vi "Log Sequence FGV.vi"(6 "Aktion":T3, 9 "Neue Gasliste gesamt":T1[](array[typedef]), 11 "Cluster (in)":T2) -> (3 "Cluster (out)":T2)   [LabVIEW 2020, in "LogKonfig.lvlib"]
uses:
  Log Sequence FGV Aktion.ctl
  Visualisierungs Elemente/String - Ausgabefeld.ctl
  LogKonfig.lvlib
  AK-Schnittstelle/AK-Schnittstelle.lvlib
  Allgemein/allgemeine Sub-VIs.lvlib
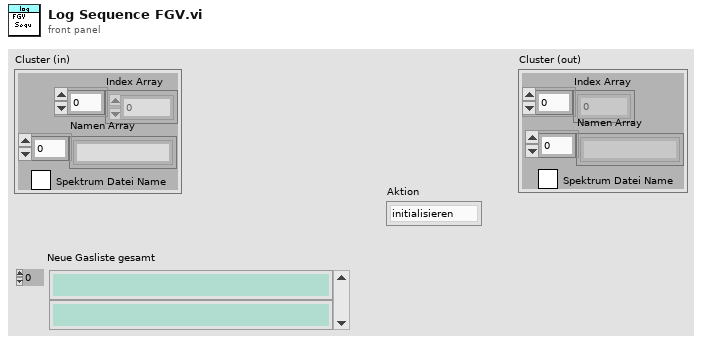
[diagram p1: front panel]
types:
  T1 = typedef "String - Ausgabefeld.ctl" = string
  T2 = cluster{"Index Array":i32[], "Namen Array":string[], "Spektrum File Name":bool}
  T3 = typedef "LogKonfig.lvlib/Log Sequence FGV Aktion.ctl" = enum16{"initialisieren", "lesen", "schreiben", "laden", "speichern", "übertragen"}
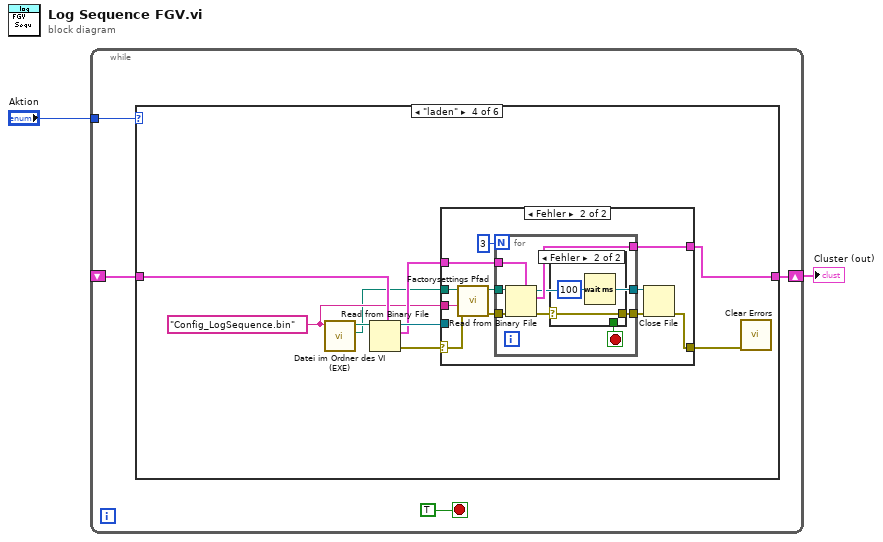
[diagram p0: block diagram]
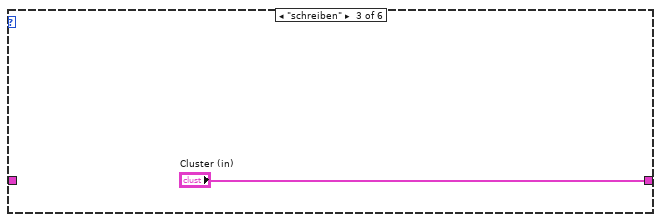
[diagram p4: hidden frame]
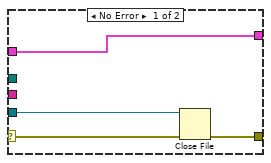
[diagram p5: hidden frame]
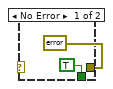
[diagram p6: hidden frame]
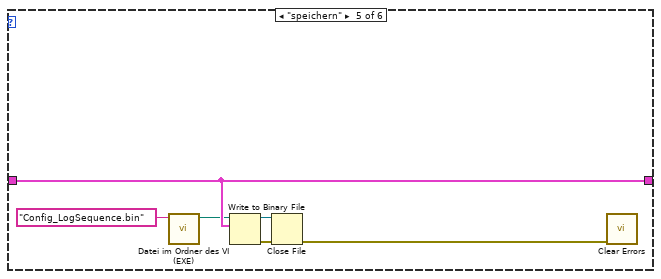
[diagram p7: hidden frame]
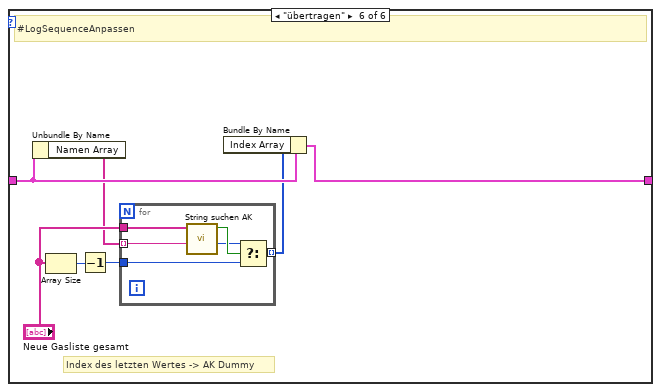
[diagram p8: hidden frame]
diagram:
  n1 = while {
    tunnel: "Aktion" -> [w5]
    shift-right: [w4] -> w1
    shift-left: _ -> [w3]
    stop <- TRUE stop-if-true
    n2 = case shown="\"laden\"" w5 {
      tunnel: [_ w7 "Cluster (in)" w13 w50 w56] -> w4
      tunnel: w3 -> [_ w7 _ w17 w50 w57]
      frame "initialisieren", Default {
      }
      frame "lesen" {
      }
      frame "schreiben" {
      }
      frame "laden" {
        w10 = "Config_LogSequence.bin" ("Dateiname")
        n3 = call "Datei im Ordner des VI (EXE).vi"("Dateiname"=w10) -> ("Ordner des Haupt-VIs"=w9:path, "Dateipfad im Ordner des Haupt-VIs"=w11:path)  [unwired: 8 in, 1 out]
        n4 = Read from Binary File(5:w17, 11:w11) -> (0:w15:errorcluster, 2:w14:T2, 3:w16:refnum<file>)  [unwired: 4 in, 1 out]
        n5 = case shown="Fehler" w15 {
          selector: w15 -> [w20 w24]
          tunnel: w14 -> [w21 w27]
          tunnel: [w21 w31] -> w13
          tunnel: [w18 w29] -> w12
          tunnel: w16 -> [w19 _]
          tunnel: w9 -> [_ w23]
          tunnel: w10 -> [_ w22]
          frame No Error {
            n6 = Close File(refnum=w19, error in=w20) -> (error out=w18:errorcluster)  [unwired: 1 out]
          }
          frame Error {
            n7 = call "Factorysettings Pfad.vi"("error in (no error)"=w24, "Dateiname"=w22, "Ordner des Haupt-VIs"=w23) -> ("error out"=w25:errorcluster, "Pfad Factorysettings"=w26:path)  [unwired: 7 in]
            n8 = for {
              N: 3 -> [_]
              tunnel: w25 -> [w38]
              tunnel: w26 -> [w37]
              tunnel: [w36] -> w31
              tunnel: [w35] -> w30
              tunnel: [w34] -> w28
              tunnel: w27 -> [w33]
              stop <- w39 stop-if-true
              n9 = Read from Binary File(5:w33, 8:w38, 11:w37) -> (0:w40:errorcluster, 2:w36:T2, 3:w34:refnum<file>)  [unwired: 3 in, 1 out]
              n10 = case shown="Fehler" w40 {
                selector: w40 -> [_ w43]
                tunnel: [TRUE _] -> w39
                tunnel: [errorcluster {"status"=FALSE, "code"=0, "source"=""} ("error IO") w43] -> w35
                frame No Error {
                }
                frame Error {
                  n11 = Wait (ms)(milliseconds to wait=u32 100 ("Zu wartende ms")) -> ()  [unwired: 1 out]
                }
              }
            }
            n12 = Close File(refnum=w28, error in=w30) -> (error out=w29:errorcluster)  [unwired: 1 out]
          }
        }
        n13 = call <vilib>:"Clear Errors.vi"("error in (no error)"=w12) -> ()  [unwired: 5 in, 2 out]
      }
      frame "speichern" {
        n14 = call "Datei im Ordner des VI (EXE).vi"("Dateiname"="Config_LogSequence.bin") -> ("Dateipfad im Ordner des Haupt-VIs"=w45:path)  [unwired: 8 in, 2 out]
        n15 = Write to Binary File(file (use dialog)=w45, data=w50) -> (refnum out=w48:refnum<file>, error out=w47:errorcluster)  [unwired: 4 in, 1 out]
        n16 = Close File(refnum=w48, error in=w47) -> (error out=w46:errorcluster)  [unwired: 1 out]
        n17 = call <vilib>:"Clear Errors.vi"("error in (no error)"=w46) -> ()  [unwired: 5 in, 2 out]
      }
      frame "übertragen" {
        # "Index des letzten Wertes -> AK Dummy"
        # "#LogSequenceAnpassen"
        n18 = Unbundle By Name(w57) -> ("Namen Array"=w52:string[])
        n19 = Array Size(array="Neue Gasliste gesamt") -> (size(s)=w55:i32)
        n20 = Decrement(x=w55) -> (x-1=w54:i32)
        n21 = for {
          tunnel: w54 -> [w60]
          tunnel: "Neue Gasliste gesamt" -> [w63]
          tunnel: w52 -> [w58] mode=indexing
          tunnel: [w59] -> w51 mode=indexing
          n22 = call "String suchen AK.vi"("gesucht"=w58, "Namen"=w63) -> ("Index"=w61:i32, "Gefunden?"=w62:bool)  [unwired: 8 in]
          n23 = Select(t=w61, s=w62, f=w60) -> (s? t:f=w59:i32)
        }
        n24 = Bundle By Name(cluster=w57, "Index Array"=w51) -> (w56:T2)
      }
    }
  }
  "Cluster (out)" <- w1
